vi "prompt_queryformation.vi"(8 "error in (no error)":errorcluster, 11 "agent_simple_qa in":refnum<class "agent_simple_qa.lvclass">) -> (0 "error out":errorcluster, 3 "agent_simple_qa out":refnum<class "agent_simple_qa.lvclass">)   [LabVIEW 2020, in "agent_simple_qa.lvclass"]
uses:
  agent_simple_qa.lvclass
  agent_simple_qa.lvclass/agent_simple_qa.ctl
  models/message_text/create_text_message.vi
  models/message_text/message_text.lvclass
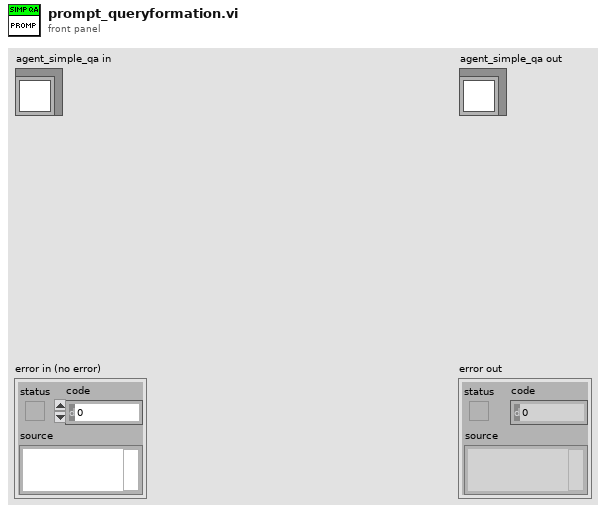
[diagram p1: front panel]
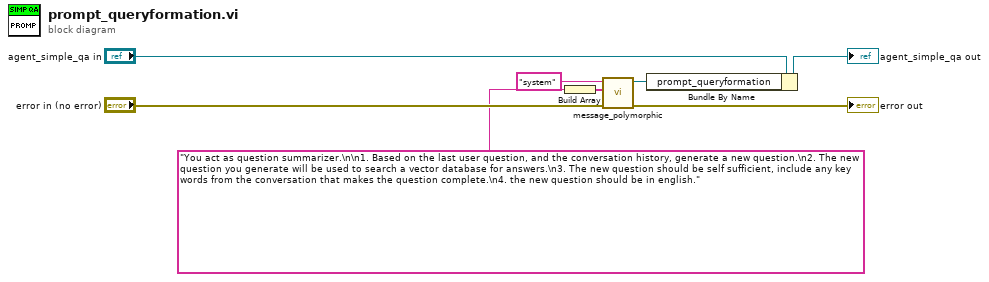
[diagram p0: block diagram]
diagram:
  n1 = Build Array("You act as question summarizer.\n\n1. Based on the last user question, and the conversation history, generate a new question.\n2. The new question you generate will be used to search a vector database for answers.\n3. The new question should be self sufficient, include any key words from the conversation that makes the question complete.\n4. the new question should be in english.") -> (w2:string[])
  n2 = call-poly "message_polymorphic.vi"("error in (no error)"="error in (no error)", "content"=w2, "role"="system") -> ("error out"=→"error out":errorcluster, "message_text out"=w3:refnum<class "message_text.lvclass">)  [unwired: 7 in]
  n3 = Bundle By Name(cluster="agent_simple_qa in", "prompt_queryformation"=w3) -> (→"agent_simple_qa out":refnum<class "agent_simple_qa.lvclass">)
